vi "Pause.vi"(8 "error in (no error)":errorcluster, 10 "Internal?":bool, 11 "Huber Settings In":T1) -> (0 "error out":errorcluster, 3 "Huber Settings Out":T1)   [LabVIEW 2021, in "Lauda TCU.lvlib"]
uses:
  Lauda TCU.lvlib
  Lauda Settings.ctl
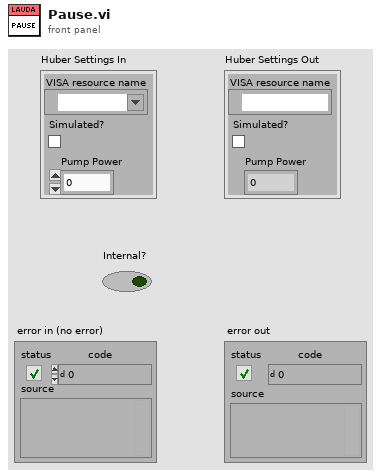
[diagram p1: front panel]
types:
  T1 = typedef "Lauda TCU.lvlib/Lauda Settings.ctl" = cluster{"VISA resource name":refnum<visa-resource-name>, "Simulated?":bool, "Pump Power":i32}
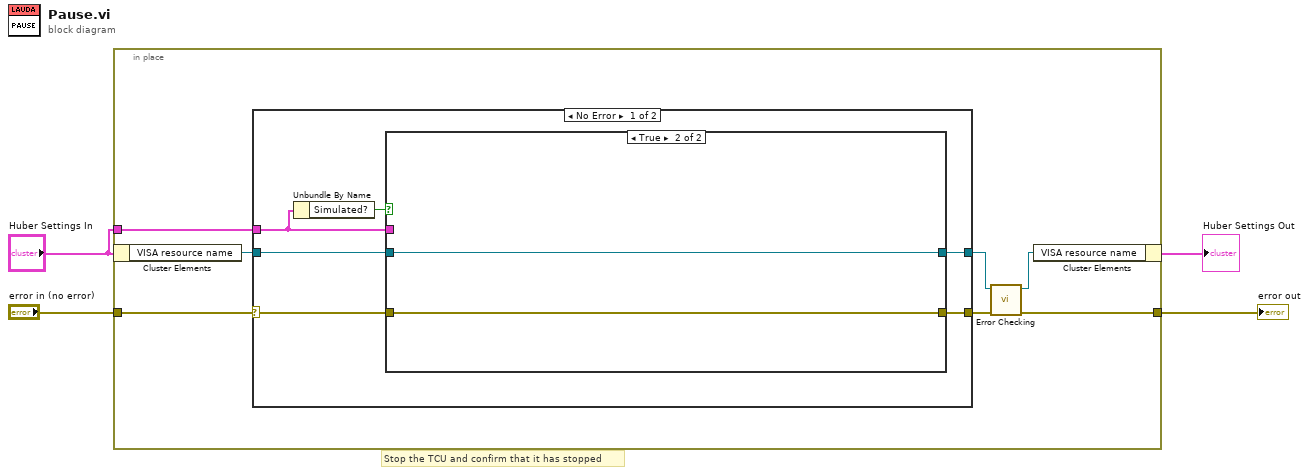
[diagram p0: block diagram]
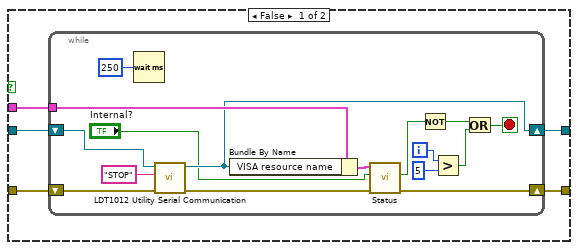
[diagram p2: hidden frame]
diagram:
  # "Stop the TCU and confirm that it has stopped"
  n1 = in-place {
    in-place-border: "error in (no error)" -> [w11]
    in-place-border: [w8] -> w3
    in-place-border: "Huber Settings In" -> [w7]
    n2 = in-place-cluster #1("Huber Settings In") -> ("VISA resource name"=w6:refnum<visa-resource-name>)
    n3 = case shown="No Error" w11 {
      selector: w11 -> [w17 w42]
      tunnel: w7 -> [w13 _]
      tunnel: [w16 w42] -> w9
      tunnel: [w15 w41] -> w10
      tunnel: w6 -> [w12 w41]
      frame No Error {
        n4 = Unbundle By Name(w13) -> ("Simulated?"=w14:bool)
        n5 = case shown="True" w14 {
          tunnel: w17 -> [w20 w40]
          tunnel: [w18 w40] -> w16
          tunnel: [w22 w39] -> w15
          tunnel: w12 -> [w21 w39]
          tunnel: w13 -> [w19 _]
          frame False {
            n6 = while {
              tunnel: w19 -> [w26]
              shift-right: [w24] -> w22
              shift-left: w21 -> [w28]
              shift-right: [w38] -> w18
              shift-left: w20 -> [w27]
              i -> [w36]
              stop <- w37 stop-if-true
              n7 = Wait (ms)(milliseconds to wait=u32 250) -> ()  [unwired: 1 out]
              n8 = call "LDT1012 Utility Serial Communication.vi"("error in (no error)"=w27, "Command String"="STOP", "VISA session"=w28) -> ("error out"=w29:errorcluster, "dup VISA session"=w24:refnum<visa-resource-name>)  [unwired: 5 in, 2 out]
              n9 = Bundle By Name(cluster=w26, "VISA resource name"=w24) -> (w25:T1)
              n10 = call "Status.vi"("error in (no error)"=w29, "Internal?"="Internal?", "Lauda Settings"=w25) -> ("error out"=w38:errorcluster, "Running"=w32:bool)  [unwired: 2 in, 5 out]
              n11 = Not(x=w32) -> (.not. x?=w31:bool)
              n12 = Greater?(x=w36, y=5) -> (0:w34:bool)
              n13 = Or(x=w31, y=w34) -> (x .or. y?=w37:bool)
            }
          }
          frame True {
          }
        }
      }
      frame Error {
      }
    }
    n14 = call "Error Checking.vi"("error in (no error)"=w9, "VISA resource name"=w10) -> ("error out"=w8:errorcluster, "VISA resource name"=w5:refnum<visa-resource-name>)  [unwired: 7 in, 1 out]
    n15 = in-place-cluster #1("VISA resource name"=w5) -> (→"Huber Settings Out":T1)
  }
  "error out" <- w3
